vi "Helmholtz2D_Cal RHS_F Inner.vi"(10 "Domain":T1={"x"={"start x"=0.0, "end x"=1.0, "# of x-points"=11}, "y"={"start y"=0.0, "end y"=1.0, "# of y-points"=11}}, 11 "F(x, y)":dbl[][](array[numeric])) -> (3 "F Inner":dbl[](array[numeric]))   [LabVIEW 2020, in "NI_PDE.lvlib"]
uses:
  <vilib>/gmath/NI_PDE.lvlib
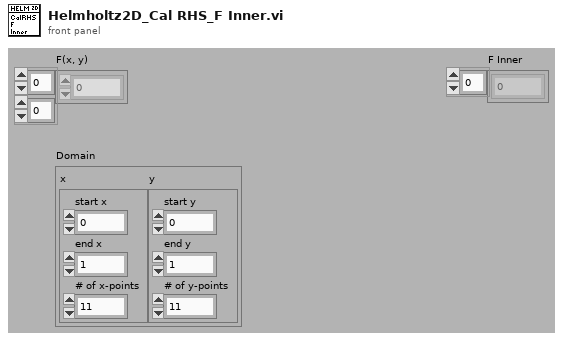
[diagram p1: front panel]
types:
  T1 = cluster{"x":cluster{"start x":dbl, "end x":dbl, "# of x-points":i32}, "y":cluster{"start y":dbl, "end y":dbl, "# of y-points":i32}}
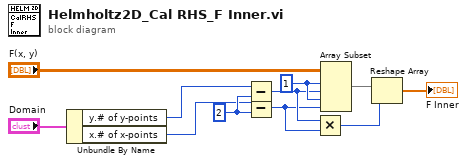
[diagram p0: block diagram]
diagram:
  w9 = 2 ("y")
  w10 = 1 ("index")
  n1 = Unbundle By Name("Domain") -> ("y.# of y-points"=w3:i32, "x.# of x-points"=w2:i32)
  n2 = Subtract(x=w3, y=w9) -> (x-y=w7:i32)
  n3 = Subtract(x=w2, y=w9) -> (x-y=w6:i32)
  n4 = Multiply(x=w7, y=w6) -> (x*y=w5:i32)
  n5 = Array Subset(array="F(x, y)", index (row)=w10, length (row)=w7, index (col)=w10, length (col)=w6) -> (w8:dbl[][])
  n6 = Reshape Array(w8, w5) -> (→"F Inner":dbl[])
